vi "subTriWave.vi"(2 "Tri Phase (s)":dbl, 3 "Sampling frequency (Hz)":dbl, 4 "Tri Repeats":dbl, 5 "Frequency":dbl, 6 "Amplitude (V)":dbl, 7 "Offset (V)":dbl) -> (0 "wfsize":i32, 1 "signal out":waveform(dbl))   [LabVIEW 2015]
uses:
  <vilib>/measure/NI_MABase.lvlib
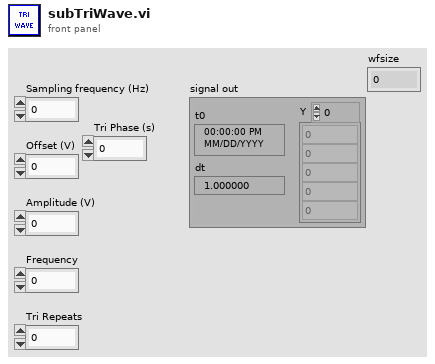
[diagram p1: front panel]
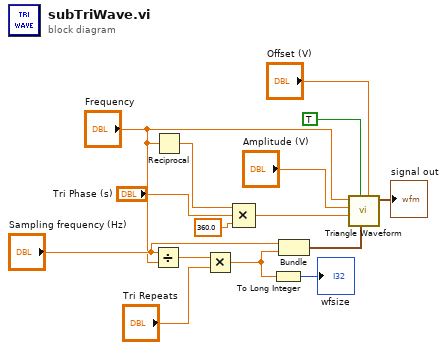
[diagram p0: block diagram]
diagram:
  n1 = Divide(x="Sampling frequency (Hz)", y="Frequency") -> (x/y=w10:dbl)
  n2 = Reciprocal(x="Frequency") -> (1/x=w9:dbl)
  n3 = Multiply(x=w10, y="Tri Repeats") -> (x*y=w2:dbl)
  n4 = Compound Arithmetic op=MULTIPLY(w9, "Tri Phase (s)", 360.0 ("value")) -> (w5:dbl)
  n5 = To Long Integer(number=w2) -> (32bit integer=→"wfsize":i32)
  n6 = Bundle("Sampling frequency (Hz)"="Sampling frequency (Hz)", w2) -> (w12:cluster{"Sampling frequency (Hz)":dbl, dbl})  [unwired: 1 in]
  n7 = call <vilib>:"Triangle Waveform.vi"("offset"="Offset (V)", "sampling info"=w12, "reset signal"=TRUE, "phase"=w5, "amplitude"="Amplitude (V)", "frequency"="Frequency") -> ("signal out"=→"signal out":waveform(dbl))  [unwired: 4 in, 1 out]
